vi "DSF.Shared.Configuration.Cycle Timed.Set Cycle Timing Factors.vi"(8 "error in (no error)":errorcluster, 10 "Cycle Timing Factors":T1={"Decimation"=1, "Offset"=0}, 11 "Cycle Timed Configuration in":refnum<class "DSF.Shared.Configuration.Cycle Timed.lvclass">) -> (0 "error out":errorcluster, 3 "Cycle Timed Configuration out":refnum<class "DSF.Shared.Configuration.Cycle Timed.lvclass">)   [LabVIEW 2016, in "DSF.Shared.lvlib" / "DSF.Shared.Configuration.Cycle Timed.lvclass"]
uses:
  DSF.Shared.Configuration.Cycle Timed.lvclass
  Typedefs/DSF.Shared.Typedefs.Cycle Timing Factors.ctl
  DSF.Shared.lvlib
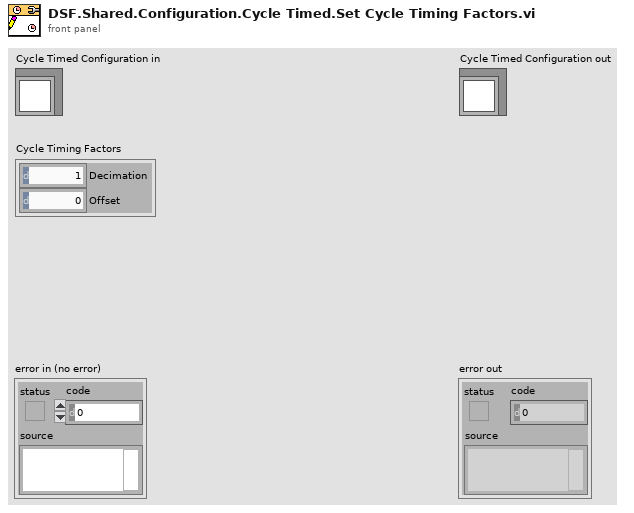
[diagram p1: front panel]
types:
  T1 = typedef "DSF.Shared.lvlib/DSF.Shared.Typedefs.Cycle Timing Factors.ctl" = cluster{"Decimation":u64, "Offset":u64}
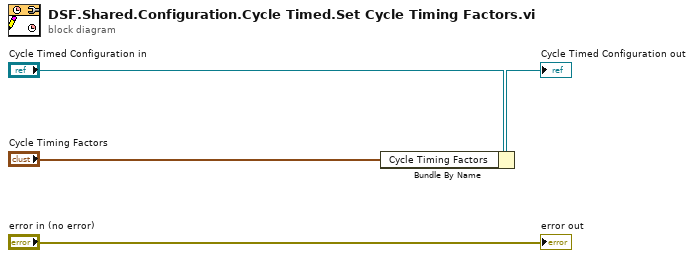
[diagram p0: block diagram]
diagram:
  n1 = Bundle By Name(cluster="Cycle Timed Configuration in", "Cycle Timing Factors"="Cycle Timing Factors") -> (→"Cycle Timed Configuration out":refnum<class "DSF.Shared.Configuration.Cycle Timed.lvclass">)
  "error out" <- "error in (no error)"
